vi "Direct Message Recieved.vi"(8 "error in (no error)":errorcluster, 10 "Message":T1, 11 "Server in":refnum<class "Server.lvclass">) -> (0 "error out":errorcluster, 3 "Server out":refnum<class "Server.lvclass">)   [LabVIEW 2015, in "Server.lvlib" / "Server.lvclass"]
uses:
  Server.lvclass
  Chat Window Model/Chat Window Model Messages/New Message Msg/New Message Msg.lvclass
  Controls/Message Control.ctl
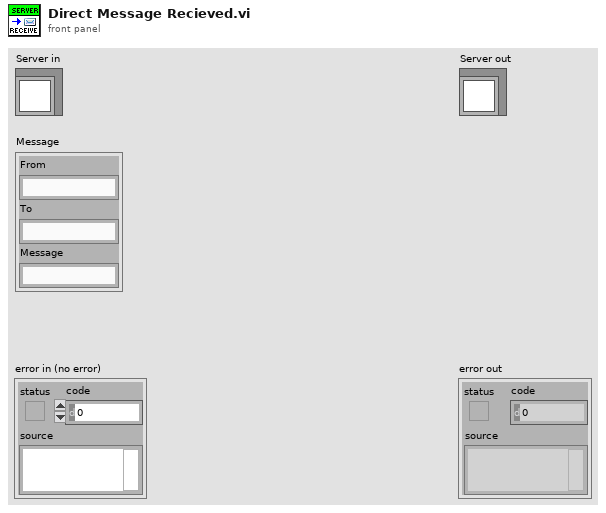
[diagram p1: front panel]
types:
  T1 = typedef "Message Control.ctl" = cluster{"From":string, "To":string, "Message":string}
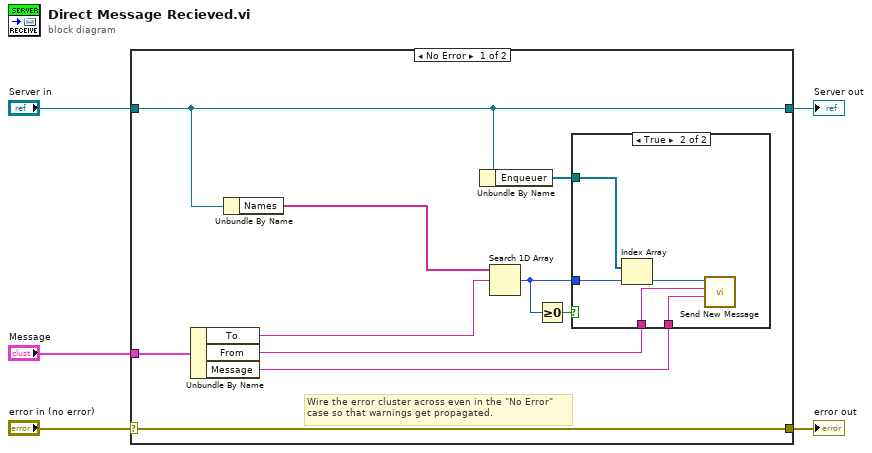
[diagram p0: block diagram]
diagram:
  n1 = case shown="No Error" "error in (no error)" {
    selector: "error in (no error)" -> [w15 w22]
    tunnel: [w15 w22] -> w4
    tunnel: [w13 w21] -> w2
    tunnel: "Server in" -> [w13 w21]
    tunnel: "Message" -> [w10 _]
    frame No Error {
      # "Wire the error cluster across even in the \"No Error\"\ncase so that warnings get propagated."
      n2 = Unbundle By Name(w10) -> ("To"=w7:string, "From"=w9:string, "Message"=w8:string)
      n3 = Unbundle By Name(w13) -> ("Names"=w6:string[])
      n4 = Unbundle By Name(w13) -> ("Enqueuer"=w12:refnum<class "Message Enqueuer.lvclass">[])
      n5 = Search 1D Array(1D array=w6, element=w7) -> (index of element=w11:i32)  [unwired: 1 in]
      n6 = Greater Or Equal To 0?(x=w11) -> (x >= 0?=w14:bool)
      n7 = case shown="True" w14 {
        tunnel: w12 -> [_ w20]
        tunnel: w11 -> [_ w19]
        tunnel: w9 -> [_ w17]
        tunnel: w8 -> [_ w16]
        frame False {
        }
        frame True {
          n8 = Index Array(array=w20, index=w19) -> (element=w18:refnum<class "Message Enqueuer.lvclass">)
          n9 = call "Send New Message.vi"("New Message"=w16, "From"=w17, "Message Enqueuer"=w18) -> ()  [unwired: 7 in, 2 out]
        }
      }
    }
    frame Error {
    }
  }
  "error out" <- w4
  "Server out" <- w2
